vi "SwissSPAD Live.vi"() -> ()   [LabVIEW 2021]
uses:
  SwissSPAD Live_Internal Variables.ctl
  <vilib>/vision/Image Controls.llb/IMAQ Image.ctl
  SwissSPAD Live_Image ROI Information.ctl
  Phasor/Image Binning Options.ctl
  SwissSPAD Live_SSx PCB Version.ctl
  SwissSPAD Live_Q [Element].ctl
  SwissSPAD Live_Q Event List.ctl
  SwissSPAD Live_Windows List.ctl
  Sound/System Sounds List.ctl
  Image/Image Display to Clipboard Options.ctl
  Image/Image Display Palette Information.ctl
  Image/Image Display Palette Type.ctl
  SwissSPAD Live_Internal Data List.ctl
  SwissSPAD Live_Globals.vi
  D:/UCLA Thinkpad Google Drive/LabVIEW 2021 SP1/builds/SwissSPAD Live Distribution/Opal Kelly/C# Wrapper/v5.0.2/libFrontPanel-csharp.dll
  Opal Kelly/C# Wrapper/v5.0.2/libFrontPanel-csharp.dll
  Notebook/Notebook.lvlib
  Rich Text Box/Rich Text Box.lvlib
  Variant/Variant to Data/Variant to Data.lvlib
  Opal Kelly/C# Wrapper/okFrontPanelC#Wrapper.lvlib
panel:
  in  "Refresh":bool
  out "Top FPGA Status":bool caption="Top"
  out "Bottom FPGA Status":bool caption="Bot"
  out "Image":T1(plugin-control)
  out "Saving in progress":bool
  in  "Animated Busy Icon":bool=TRUE
  in  "Record Button":bool
  in  "Live Button":bool
  in  "Abort":bool
  out "Message":string
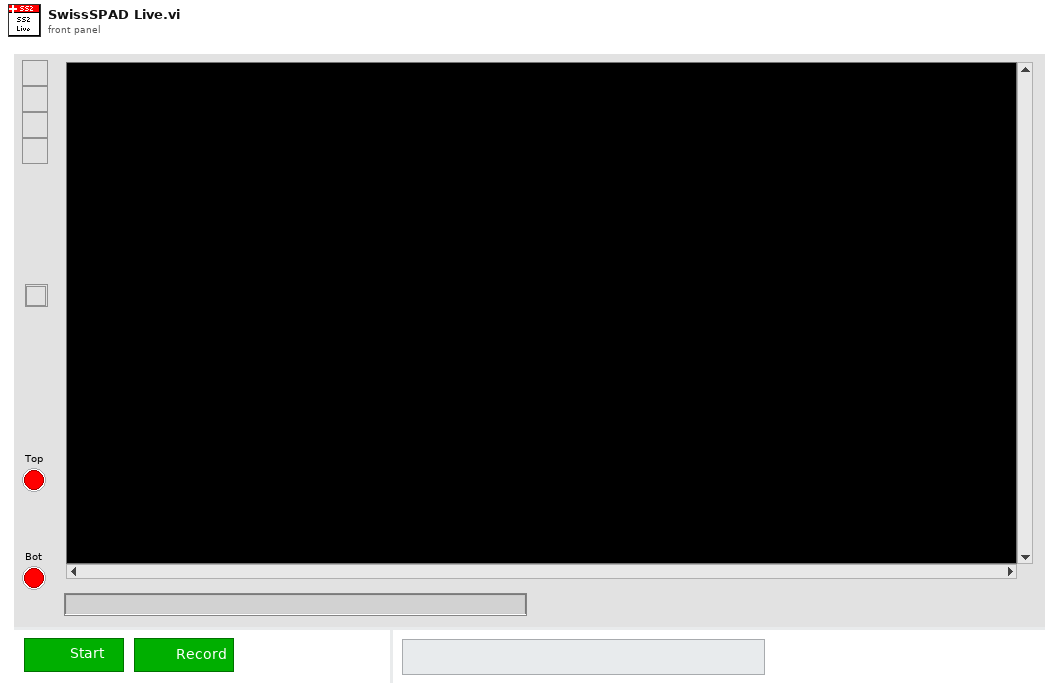
[diagram p1: front panel]
types:
  T1 = typedef "IMAQ Image.ctl" = refnum<image>
  T2 = typedef "SwissSPAD Live_Windows List.ctl" = enum16{"Settings Window", "Notebook Window", "Histogram Window", "About Window", "SS2 Live Window"}
  T3 = typedef "SwissSPAD Live_Q Event List.ctl" = enum16{"---- UI ----", "Idle", "Initialization", "Init FPGA(s)", "Init Top FPGA (deprecated)", "FPGA(s) Status", "Top FPGA Status (deprecated)", "Reset FPGA(s)", "Reset Top FPGA (deprecated)", "Refresh Display Image", "Quit", "---- DAQ ----", "Start Recording", "Start Live Acquisition", "Initialize Recording Mode", "Initialize FPGA (Live Mode)", "Get Image Set", "Get Single Image", "Update Image Display", "Stop Live Acquisition", "Stop Data Recording", "Stop Data Saving", "---- Image ----", "Copy Data to Clipboard", "Set Image Palette", "Save Displayed Image with Overlay", "Save Image Data as TIFF"}
  T4 = typedef "SwissSPAD Live_Q [Element].ctl" = cluster{"SwissSPAD Q Event":T3, "Data":variant}
  T5 = typedef "SwissSPAD Live_Internal Variables.ctl" = cluster{"okCFrontPanelDevices Refnum":refnum<k24>, "Bottom Device Refnum":refnum<k24>, "Display Image":T1, "# Live Images":i32, "relative s":dbl, "# Image Sets":i32, "Message":string, "Current Image Set":i32, "# Datasets in Series":i32, "Current Dataset":i32, "Live Mode":bool, "Recording Mode":bool, "Record Button":refnum<vi>, "\nLive Button":refnum<vi>, "SwissSPAD Live Gate Image Data Q Name":string, "Discard First Image":bool, "Image Information":T6, "Image Binning Options":T7, "Bottom FPGA Serial Number":string, "Detector PCB Version":T8, "# Acquisitions":u32, "10 bits":bool, "Top FPGA Serial Number":string, "Top Device Refnum":refnum<k24>}
  T6 = typedef "SwissSPAD Live_Image ROI Information.ctl" = cluster{"Save ROI Only":bool, "Left":u16, "Top":u16, "Right":u16, "Bottom":u16, "Use Current ROI":bool}
  T7 = typedef "Image Binning Options.ctl" = cluster{"Use Image Binning":bool, "X Bin":i32, "Y Bin":i32}
  T8 = typedef "SwissSPAD Live_SSx PCB Version.ctl" = enum16{"unknown", "SS2 PCB1", "SS2 PCB2", "SS3 PCB1"}
  T9 = typedef "System Sounds List.ctl" = enum16{"Alarm01", "Alarm02", "Alarm03", "Alarm04", "Alarm05", "Alarm06", "Alarm07", "Alarm08", "Alarm09", "Alarm10", "chimes", "chord", "ding", "notify", "recycle", "Ring01", "Ring02", "Ring03", "Ring04", "Ring05", "Ring06", "Ring07", "Ring08", "Ring09", "Ring10", "ringout", "Speech Off", "Speech On", "Speech Sleep", "tada", "Windows Background", "Windows Balloon", "Windows Battery Critical", "Windows Battery Low", "Windows Critical Stop", "Windows Default", "Windows Ding", "Windows Error", "Windows Exclamation", "Windows Feed Discovered", "Windows Foreground", "Windows Hardware Fail", "Windows Hardware Insert", "Windows Hardware Remove", "Windows Information Bar", "Windows Logoff Sound", "Windows Logon", "Windows Menu Command", "Windows Message Nudge", "Windows Minimize", "Windows Navigation Start", "Windows Notify Calendar", "Windows Notify Email", "Windows Notify Messaging", "Windows Notify System Generic", "Windows Notify", "Windows Pop-up Blocked", "Windows Print complete", "Windows Proximity Connection", "Windows Proximity Notification", "Windows Recycle", "Windows Restore", "Windows Ringin", "Windows Ringout", "Windows Shutdown", "Windows Startup", "Windows Unlock", "Windows User Account Control"}
  T10 = typedef "Image Display to Clipboard Options.ctl" = cluster{"Include Overlay (T)":bool, "Image Only (T)":bool}
  T11 = cluster{"CtlRef":refnum<vi>, "Image to Clipboard Options":T10}
  T12 = typedef "Image Display Palette Information.ctl" = cluster{"Palette Name [# Colors,int?,inv?]":string, "Palette Type":T13, "Palette Colors":u32[], "Interpolate?":bool}
  T13 = typedef "Image Display Palette Type.ctl" = u32
  T14 = typedef "SwissSPAD Live_Init Communication Outcome.ctl" = cluster{"Bottom FPGA Found":bool, "Top FPGA Found":bool, "# Orphan FPGAs":i32, "Orphaned FPGA S/N":string[]}
  T15 = typedef "Rich Text Box.lvlib/Text Formatting.ctl" = cluster{"Font":string, "Text Color":T16, "Text Background Color":T16, "Text Style":enum16{"Regular", "Bold", "Italic", "Underline", "Strikeout"}, "Font Size (Points)":dbl, "Text Alignment":i32}
  T16 = typedef "Rich Text Box.lvlib/Text Colors.ctl" = enum16{"Unchanged", "Black", "Blue", "Brown", "Gray", "Green", "Orange", "Pink", "Red", "White"}
  T17 = typedef "Save File Format.ctl" = enum16{"PNG", "JPEG", "BMP"}
  T18 = typedef "SwissSPAD Live_Internal Data List.ctl" = enum16{"Number of pending file saving tasks", "File Saving Tasks Information", "Current Image ROI Information", "# FPGA Reset Attempts", "Histogram Cursor Locations", "Histogram Window is Open"}
  T19 = cluster{"Global Rectangle":i32[], "Contours":cluster{"Contour Type":u32, "ROI Type":u32, "Points":i32[]}[]}
  T20 = typedef "SwissSPAD Live_File Saving Task Information.ctl" = cluster{"File Path::n":string, "# Saved Images":i32, "# Images (Total)":i32, "File Size (Bytes)":i64}
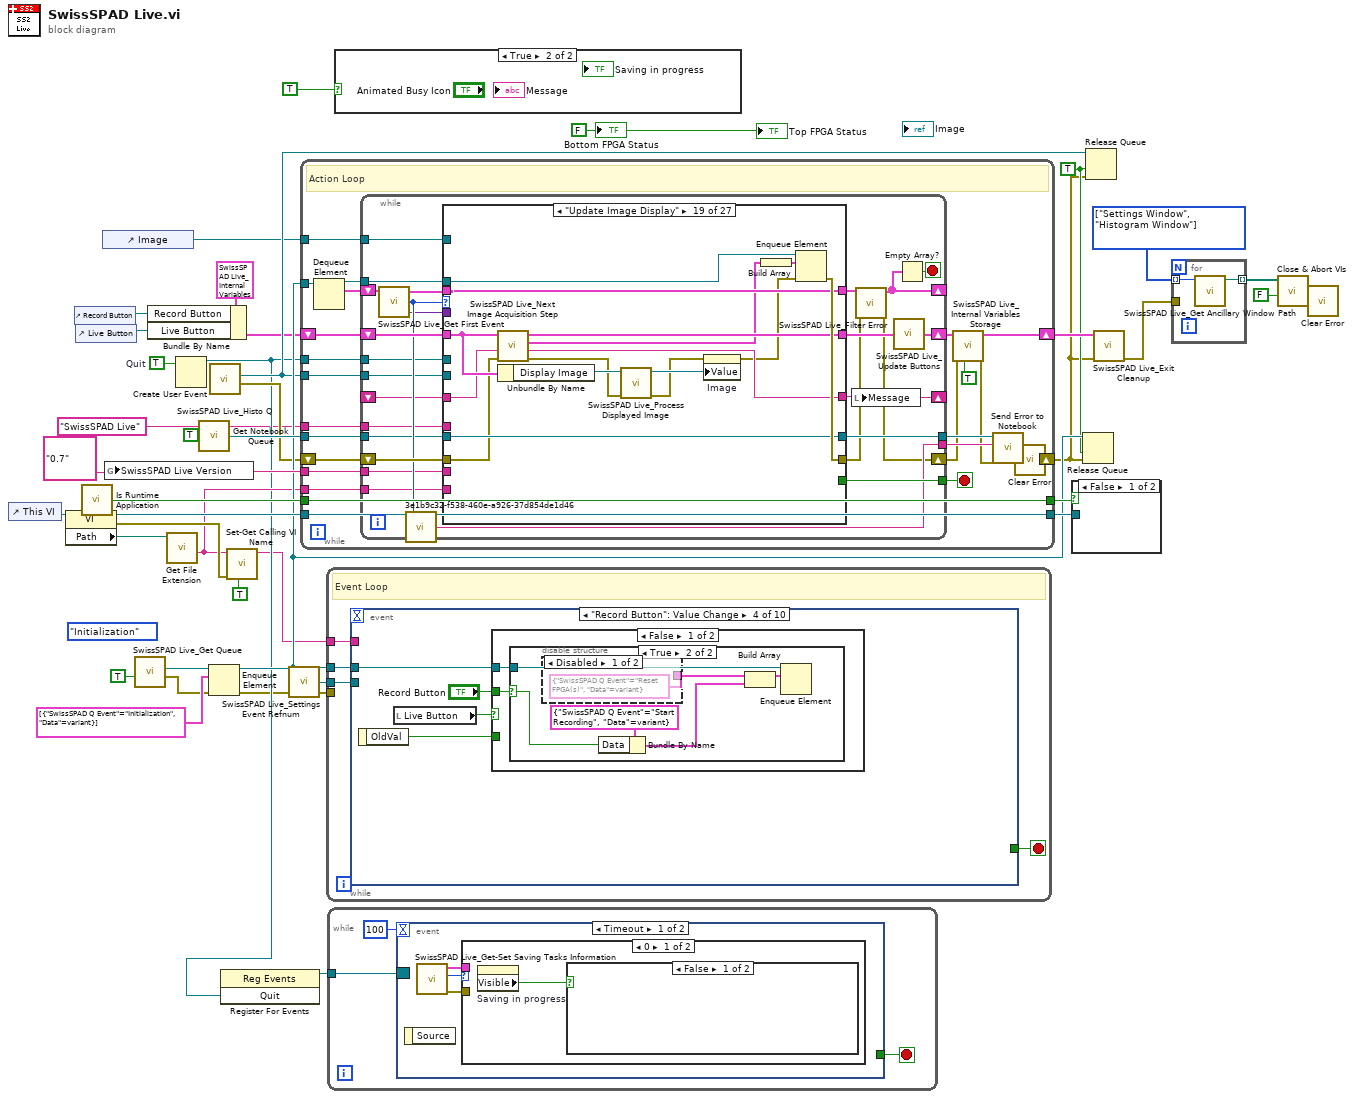
[diagram p0: block diagram]
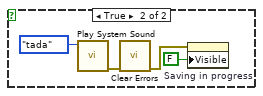
[diagram p2: hidden frame]
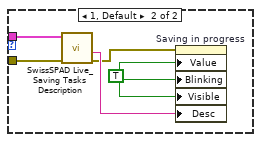
[diagram p3: hidden frame]
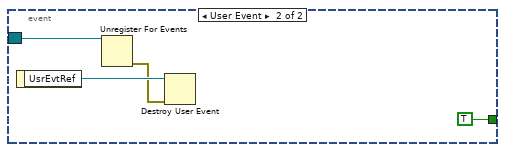
[diagram p4: hidden frame]
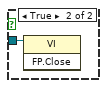
[diagram p6: hidden frame]
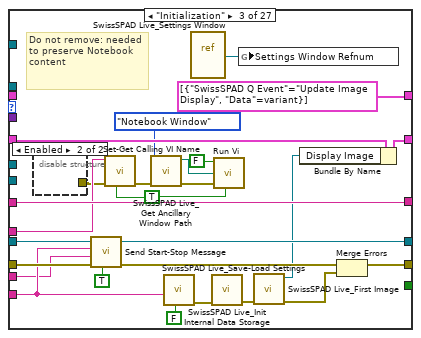
[diagram p9: hidden frame]
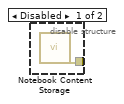
[diagram p10: hidden frame]
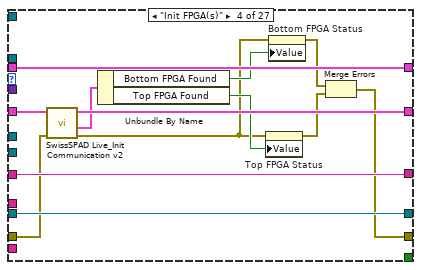
[diagram p11: hidden frame]
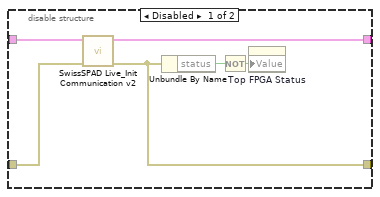
[diagram p13: hidden frame]
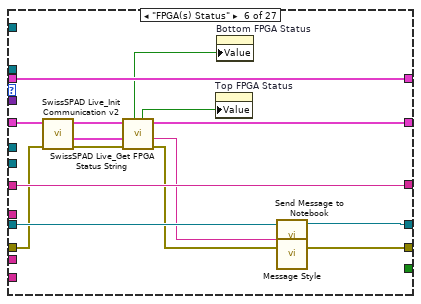
[diagram p14: hidden frame]
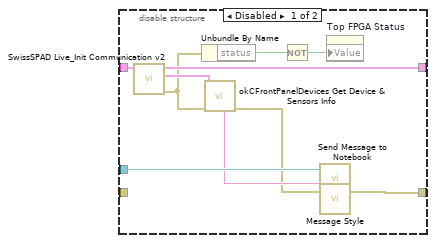
[diagram p16: hidden frame]
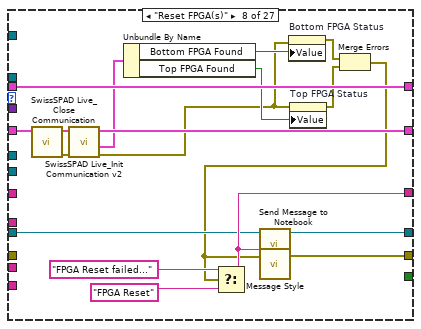
[diagram p17: hidden frame]
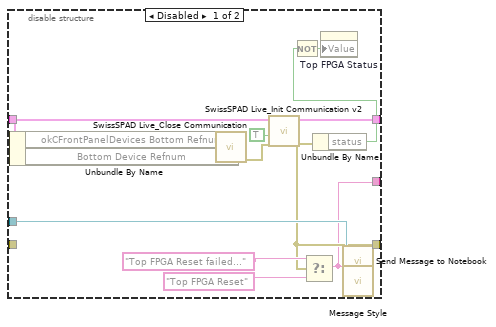
[diagram p19: hidden frame]
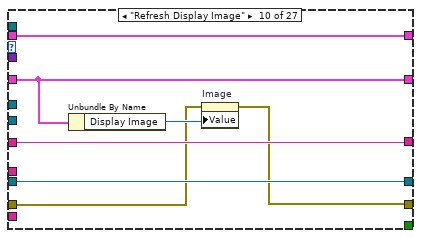
[diagram p20: hidden frame]
diagram:
  w6 = T2[] [enum."Settings Window", enum."Histogram Window"] items=["Settings Window", "Notebook Window", "Histogram Window", "About Window", "SS2 Live Window"] ("Array")
  (unwired) SwissSPAD_Live_Q_Event_List."Initialization" ("SwissSPAD Q Event")
  w7 = FALSE ("FPGA Status")
  w22 = TRUE  # Quit
  w25 = TRUE ("force destroy? (F)")
  w30 = "0.7" ("SS2 Live Version")
  n1 = control-ref of="This VI"() -> (w40:refnum<vi>)
  n2 = property class="VI"(reference=w40) -> (reference out=w37:refnum<vi>, error out=w36:errorcluster, "Path"=w26:path)  [unwired: 1 in]
  n3 = control-ref of="Record Button"() -> (w12:refnum<vi>)
  n4 = control-ref of="Live Button"() -> (w13:refnum<vi>)
  n5 = call "Is Runtime Application.vi"() -> ("Runtime ?"=w42:bool)  [unwired: 8 in, 1 out]
  n6 = control-ref of="Image"() -> (w15:refnum<vi>)
  n7 = global write "SwissSPAD Live_Globals.vi" "SwissSPAD Live Version"(w30) -> ()
  n8 = call "SwissSPAD Live_Get Queue.vi"("create if not found? (F)"=TRUE) -> ("error out"=w9:errorcluster, "SwissSPAD Queue"=w10:refnum<queue>)  [unwired: 9 in]
  n9 = Bundle By Name(cluster=T5 {"okCFrontPanelDevices Refnum"=refnum, "Bottom Device Refnum"=refnum, "Display Image"=refnum, "# Live Images"=0, "relative s"=nan, "# Image Sets"=0, "Message"="", "Current Image Set"=0, "# Datasets in Series"=0, "Current Dataset"=0, "Live Mode"=FALSE, "Recording Mode"=FALSE, "Record Button"=refnum, "\nLive Button"=refnum, "SwissSPAD Live Gate Image Data Q Name"="SS2 Live Gate Data Q", "Discard First Image"=FALSE, "Image Information"={"Save ROI Only"=FALSE, "Left"=0, "Top"=0, "Right"=0, "Bottom"=0, "Use Current ROI"=FALSE}, "Image Binning Options"={"Use Image Binning"=FALSE, "X Bin"=1, "Y Bin"=1}, "Bottom FPGA Serial Number"="", "Detector PCB Version"=enum."unknown", "# Acquisitions"=0, "10 bits"=FALSE, "Top FPGA Serial Number"="", "Top Device Refnum"=refnum}, "Record Button"=w12, "Live Button"=w13) -> (w14:T5)
  n10 = call <vilib>:"Get File Extension.vi"("file"=w26) -> ("filename without extension"=w27:string)  [unwired: 6 in, 4 out]
  n11 = Create User Event(user event datatype=w22) -> (user event=w20:refnum<user-event>)  [unwired: 1 in, 1 out]
  n12 = call "Get Notebook Queue.vi"("create if not found? (T)"=TRUE ("create if not found? (F)")) -> ("Notebook Queue"=w31:refnum<queue>)  [unwired: 8 in]
  n13 = Enqueue Element(queue=w10, element=T4[] [{"SwissSPAD Q Event"=enum."Initialization", "Data"=variant}], error in (no error)=w9) -> (queue out=w29:refnum<queue>, error out=w19:errorcluster)  [unwired: 1 in, 1 out]
  n14 = call "SwissSPAD Live_Histo Q.vi"() -> ("error out"=w24:errorcluster, "SS2 Live Histo Q"=w23:refnum<queue>)  [unwired: 6 in]
  n15 = register-events(w20) -> (reference out=w21:refnum<event-registration>)  [unwired: 2 in, 1 out]
  n16 = call "Set-Get Calling VI Name.vi"("Set/Get (F)"=TRUE, "Error In"=w36, "Calling VI Name"=w27) -> ("Calling VI Name"=w16:string)  [unwired: 7 in, 1 out]
  n17 = call "SwissSPAD Live_Settings Event Refnum.vi"("Error In"=w19) -> ("Settings Event Refnum"=w17:refnum<user-event>, "Error Out"=w18:errorcluster)  [unwired: 7 in]
  n18 = while {
    tunnel: w29 -> [w66]
    tunnel: w42 -> [w61]
    tunnel: [w61] -> w41
    tunnel: w37 -> [w60]
    tunnel: [w60] -> w39
    shift-right: [w54] -> w5
    shift-left: w24 -> [w63]
    shift-right: [w46] -> w33
    shift-left: w14 -> [w59]
    tunnel: w31 -> [w57]
    tunnel: w30 -> [w52]
    tunnel: w27 -> [w51]
    tunnel: w23 -> [w50]
    tunnel: w20 -> [w49]
    tunnel: w15 -> [w48]
    tunnel: "SwissSPAD Live" ("Calling VI Name") -> [w47]
    stop <- w64 stop-if-true
    # "Action Loop"
    n19 = Dequeue Element(queue=w66) -> (queue out=w62:refnum<queue>, element=w65:T4[])  [unwired: 2 in, 2 out]
    n20 = while {
      tunnel: [w92] -> w64
      tunnel: w62 -> [w90]
      shift-right: [w68] -> w44
      shift-left: w63 -> [w91]
      shift-right: [w67] -> _
      shift-left: w65 -> [w89]
      shift-right: [w76] -> w58
      shift-left: w59 -> [w86]
      tunnel: w57 -> [w83]
      tunnel: [w71] -> w56
      tunnel: [w84] -> w53
      tunnel: w52 -> [w82]
      tunnel: w51 -> [w81]
      shift-right: [w80] -> _
      shift-left: _ -> [w79]
      tunnel: w50 -> [w77]
      tunnel: w49 -> [w75]
      tunnel: w48 -> [w73]
      tunnel: w47 -> [w72]
      stop <- w87 stop-if-true
      n21 = call "SwissSPAD Live_Get First Event.vi"("SS2 Q Element"=w89) -> ("Data"=w78:variant, "SS2 Q Event"=w85:T3, "SS2 Q Elements"=w88:T4[])  [unwired: 2 in]
      n22 = call "3e1b9c32-f538-460e-a926-37d854de1d46.vi"("Enum"=w85) -> ("String"=w84:string)
      n23 = case shown="\"Update Image Display\"" w85 {
        tunnel: [_ _ _ _ _ _ _ _ _ _ w252 _ _ _ _ _ _ _ _ _ _ _ _ _ _ _ _] -> w92
        tunnel: w91 -> [w97 w102 w121 w136 w143 w157 w173 _ w212 w236 w253 w266 w271 w292 w303 w316 _ w356 w367 w378 _ w404 w412 w420 w425 w442 w479]
        tunnel: w90 -> [_ _ _ _ _ _ _ _ _ _ _ _ w276 w295 w307 w320 w348 w359 w372 w384 w397 _ _ _ _ _ _]
        tunnel: [w97 w102 w126 w129 w142 w169 w177 w202 w214 w235 w261 w266 w275 w286 w296 w319 w339 w353 w375 w382 w387 w401 w412 w414 w426 w447 w484] -> w70
        tunnel: w88 -> [w96 w101 _ w141 w148 w172 w179 w211 w218 w241 _ w265 w274 w293 w305 w318 w346 w358 w374 _ _ w407 w411 w424 w439 w451 w488]
        tunnel: [w96 w101 T4[] [{"SwissSPAD Q Event"=enum."Update Image Display", "Data"=variant}] ("SS2 Q Elements") w141 w148 w172 w179 w211 w218 w241 _ w265 w274 w293 w305 w318 w346 w358 w374 _ _ w407 w411 w424 w439 w451 w488] -> w69
        tunnel: w86 -> [w93 w100 w127 w138 w145 w167 w175 w200 w216 w238 w244 w262 w273 w291 w304 w311 w343 w355 w370 w379 w386 w406 w408 w419 w430 w450 w486]
        tunnel: [w93 w100 w115 w137 w144 w163 w174 w210 w217 w238 w243 w262 w273 w289 w300 w310 w342 w351 w369 w377 w395 w406 w408 w419 w430 w450 w486] -> w74
        tunnel: w77 -> [_ _ _ _ _ _ _ _ _ _ w256 _ _ _ _ _ _ _ _ _ _ _ _ _ _ _ _]
        tunnel: w83 -> [w95 w99 w123 w140 w147 w168 w176 w203 w215 w240 w254 w264 w270 w290 w301 w315 w341 w357 w373 w381 w393 w402 w410 w423 w438 w440 w483]
        tunnel: w82 -> [_ _ w119 _ _ _ _ _ _ _ w248 _ _ _ _ _ _ _ _ _ _ _ _ _ _ _ _]
        tunnel: w81 -> [_ _ w120 _ _ _ _ _ _ _ w249 _ _ _ _ _ _ _ _ _ _ _ _ _ _ _ _]
        tunnel: [w95 w99 w123 w140 w147 w164 w176 w204 w215 w240 w254 w264 w270 w290 w301 w315 w335 w357 w373 w381 w393 w398 w410 w423 w438 w440 w475] -> w71
        tunnel: [w94 w98 w125 w139 w146 w171 w178 w205 w213 w239 w259 w263 w272 w287 w297 w313 "" ("Message") w349 w366 "Live Mode stopped" ("Message") "Data Recording stopped" ("Message") w399 w409 w422 w437 w449 w487] -> w80
        tunnel: w79 -> [w94 w98 w125 w139 w146 w171 w178 _ _ w239 w259 w263 _ _ _ _ _ _ w365 _ _ _ w409 w422 w437 w449 w487]
        tunnel: w78 -> [_ _ _ _ _ _ _ _ _ _ _ _ _ _ _ w309 _ _ _ _ _ _ _ w421 w432 _ _]
        tunnel: w75 -> [_ _ _ _ _ _ _ _ _ _ w247 _ _ _ _ _ _ _ _ _ _ _ _ _ _ _ _]
        tunnel: w73 -> [_ _ _ _ _ _ _ _ _ _ _ _ _ _ _ _ _ _ _ _ _ _ _ _ w427 w448 _]
        tunnel: w72 -> [_ _ w109 _ _ _ _ _ _ _ _ _ _ _ _ _ _ _ _ _ _ _ _ _ _ _ _]
        frame "---- UI ----" {
        }
        frame "Idle", Default {
        }
        frame "Initialization" {
          w107 = TRUE ("Start Hidden? (F)")
          # "Do not remove: needed to preserve Notebook content"
          n24 = disable-structure shown="Enabled" {
            disable-tunnel: [w128 _] -> w108
            frame Disabled {
              n25 = call "Notebook Content Storage.vi"() -> ("Error Out"=w128:errorcluster)  [unwired: 10 in, 1 out]
            }
            frame Enabled {
            }
          }
          n26 = call "Send Start-Stop Message.vi"("Start(T)/Stop(F)"=TRUE ("Start(F)/Stop(T)"), "Error In"=w121, "Version number"=w119, "Software Name"=w120, "Notebook Queue"=w123) -> ("Error Out"=w122:errorcluster)  [unwired: 6 in]
          n27 = call "Set-Get Calling VI Name.vi"("Set/Get (F)"=w107, "Error In"=w108, "Calling VI Name"=w109) -> ("Error Out"=w110:errorcluster)  [unwired: 7 in, 1 out]
          n28 = call "SwissSPAD Live_Get Ancillary Window Path.vi"("Error In"=w110, "SS2 Live Windows"=SwissSPAD_Live_Windows_List."Notebook Window") -> ("Error Out"=w113:errorcluster, "VI Path"=w112:path)  [unwired: 8 in]
          n29 = call "SwissSPAD Live_Save-Load Settings.vi"("Load(F)/Save (T)"=FALSE, "App Name"=w120) -> ("Error Out"=w106:errorcluster)  [unwired: 8 in, 1 out]
          n30 = vi-ref "SwissSPAD Live_Settings Window.vi"() -> (w124:refnum<vi>)
          n31 = call "SwissSPAD Live_Init Internal Data Storage.vi"("Error In"=w106) -> ("Error Out"=w104:errorcluster)  [unwired: 10 in]
          n32 = call "Run Vi.vi"("Bring To Front (T)"=FALSE, "VI Path"=w112, "error in (no error)"=w113, "Start Hidden? (F)"=w107) -> ()  [unwired: 4 in, 2 out]
          n33 = global write "SwissSPAD Live_Globals.vi" "Settings Window Refnum"(w124) -> ()
          n34 = call "SwissSPAD Live_First Image.vi"("error in"=w104) -> ("error out"=w103:errorcluster, "Image"=w114:T1)  [unwired: 9 in]
          n35 = Bundle By Name(cluster=w127, "Display Image"=w114) -> (w115:T5)
          n36 = Merge Errors(w122, w103) -> (w126:errorcluster)
        }
        frame "Init FPGA(s)" {
          n37 = call "SwissSPAD Live_Init Communication v2.vi"("Error In"=w136, "SwissSPAD Live Internal Variables in"=w138) -> ("Error Out"=w132:errorcluster, "Init Communication Outcome"=w135:T14, "SwissSPAD Live Internal Variables out"=w137:T5)  [unwired: 7 in]
          n38 = Unbundle By Name(w135) -> ("Bottom FPGA Found"=w134:bool, "Top FPGA Found"=w133:bool)
          n39 = property on="Top FPGA Status" class="Bool (strict)"(error in=w132, "Value"=w133) -> (error out=w130:errorcluster)  [unwired: 1 in, 1 out]
          n40 = property on="Bottom FPGA Status" class="Bool (strict)"(error in=w132, "Value"=w134) -> (error out=w131:errorcluster)  [unwired: 1 in, 1 out]
          n41 = Merge Errors(w131, w130) -> (w129:errorcluster)
        }
        frame "Init Top FPGA (deprecated)" {
          n42 = disable-structure shown="Enabled" {
            disable-tunnel: w145 -> [w154 w156]
            disable-tunnel: [w153 w156] -> w144
            disable-tunnel: w143 -> [w152 w155]
            disable-tunnel: [w151 w155] -> w142
            frame Disabled {
              n43 = call "SwissSPAD Live_Init Communication v2.vi"("Error In"=w152, "SwissSPAD Live Internal Variables in"=w154) -> ("Error Out"=w151:errorcluster, "SwissSPAD Live Internal Variables out"=w153:T5)  [unwired: 7 in, 1 out]
              n44 = Unbundle By Name(w151) -> ("status"=w150:bool)
              n45 = Not(x=w150) -> (.not. x?=w149:bool)
              n46 = property on="Top FPGA Status" class="Bool (strict)"("Value"=w149) -> ()  [unwired: 2 in, 2 out]
            }
            frame Enabled {
            }
          }
        }
        frame "FPGA(s) Status" {
          n47 = call "SwissSPAD Live_Init Communication v2.vi"("Error In"=w157, "SwissSPAD Live Internal Variables in"=w167) -> ("Error Out"=w165:errorcluster, "Init Communication Outcome"=w161:T14, "SwissSPAD Live Internal Variables out"=w160:T5)  [unwired: 7 in]
          n48 = call "SwissSPAD Live_Get FPGA Status String.vi"("error in (no error)"=w165, "Init Communication Outcome"=w161, "SwissSPAD Live Internal Variables in"=w160) -> ("error out"=w166:errorcluster, "Device Info String"=w162:string, "SwissSPAD Live Internal Variables out"=w163:T5, "Top FPGA Status"=w158:bool, "Bottom FPGA Status"=w159:bool)  [unwired: 4 in]
          n49 = property on="Top FPGA Status" class="Bool (strict)"("Value"=w158) -> ()  [unwired: 2 in, 2 out]
          n50 = property on="Bottom FPGA Status" class="Bool (strict)"("Value"=w159) -> ()  [unwired: 2 in, 2 out]
          n51 = call "Message Style.vi"() -> ("Message Formatting"=w170:T15)
          n52 = call "Send Message to Notebook.vi"("Text Formatting"=w170, "Error In"=w166, "Message"=w162, "Notebook Queue"=w168) -> ("Error Out"=w169:errorcluster, "Notebook Queue"=w164:refnum<queue>)  [unwired: 4 in]
        }
        frame "Top FPGA Status (deprecated)" {
          n53 = disable-structure shown="Enabled" {
            disable-tunnel: [w189 w191] -> w177
            disable-tunnel: w176 -> [w188 _]
            disable-tunnel: w175 -> [w187 w192]
            disable-tunnel: [w183 w192] -> w174
            disable-tunnel: w173 -> [_ w191]
            frame Disabled {
              n54 = call "SwissSPAD Live_Init Communication v2.vi"("SwissSPAD Live Internal Variables in"=w187) -> ("Error Out"=w182:errorcluster, "Init Communication Outcome"=w186:T14, "SwissSPAD Live Internal Variables out"=w183:T5)  [unwired: 8 in]
              n55 = Unbundle By Name(w182) -> ("status"=w181:bool)
              n56 = call "okCFrontPanelDevices Get Device & Sensors Info.vi"("error in (no error)"=w182, "okCFrontPanel Device Refnum"=w186) -> ("error out"=w184:errorcluster, "Device Info String"=w185:string)  [unwired: 5 in, 3 out]
              n57 = Not(x=w181) -> (.not. x?=w180:bool)
              n58 = call "Message Style.vi"() -> ("Message Formatting"=w190:T15)
              n59 = call "Send Message to Notebook.vi"("Text Formatting"=w190, "Error In"=w184, "Message"=w185, "Notebook Queue"=w188) -> ("Error Out"=w189:errorcluster)  [unwired: 7 in]
              n60 = property on="Top FPGA Status" class="Bool (strict)"("Value"=w180) -> ()  [unwired: 2 in, 2 out]
            }
            frame Enabled {
            }
          }
        }
        frame "Reset FPGA(s)" {
          n61 = call "SwissSPAD Live_Close Communication.vi"("SwissSPAD Live Internal Variables"=w200) -> ("Error Out"=w209:errorcluster, "SwissSPAD Live Internal Variables"=w201:T5)  [unwired: 9 in]
          n62 = call "SwissSPAD Live_Init Communication v2.vi"("Error In"=w209, "SwissSPAD Live Internal Variables in"=w201) -> ("Error Out"=w196:errorcluster, "Init Communication Outcome"=w199:T14, "SwissSPAD Live Internal Variables out"=w210:T5)  [unwired: 7 in]
          n63 = Unbundle By Name(w199) -> ("Bottom FPGA Found"=w198:bool, "Top FPGA Found"=w197:bool)
          n64 = call "Message Style.vi"() -> ("Message Formatting"=w208:T15)
          n65 = property on="Bottom FPGA Status" class="Bool (strict)"(error in=w196, "Value"=w198) -> (error out=w195:errorcluster)  [unwired: 1 in, 1 out]
          n66 = property on="Top FPGA Status" class="Bool (strict)"(error in=w196, "Value"=w197) -> (error out=w193:errorcluster)  [unwired: 1 in, 1 out]
          n67 = Merge Errors(w195, w193) -> (w194:errorcluster)
          n68 = Select(t="FPGA Reset failed...", s=w194, f="FPGA Reset" ("UI Message")) -> (s? t:f=w205:string)
          n69 = call "Send Message to Notebook.vi"("Text Formatting"=w208, "Error In"=w194, "Message"=w205, "Notebook Queue"=w203) -> ("Error Out"=w202:errorcluster, "Notebook Queue"=w204:refnum<queue>)  [unwired: 4 in]
        }
        frame "Reset Top FPGA (deprecated)" {
          n70 = disable-structure shown="Enabled" {
            disable-tunnel: [w232 w234] -> w217
            disable-tunnel: w216 -> [w229 w234]
            disable-tunnel: w215 -> [w225 _]
            disable-tunnel: [w222 w233] -> w214
            disable-tunnel: [w219 _] -> w213
            disable-tunnel: w212 -> [_ w233]
            frame Disabled {
              n71 = Unbundle By Name(w229) -> ("okCFrontPanelDevices Bottom Refnum"=w231:refnum<k24>, "Bottom Device Refnum"=w230:refnum<k24>)
              n72 = call "SwissSPAD Live_Close Communication.vi"(10:w230, "SwissSPAD Live Internal Variables"=w231) -> ("Error Out"=w228:errorcluster)  [unwired: 8 in, 1 out]
              n73 = call "SwissSPAD Live_Init Communication v2.vi"("Init Communication Outcome"=TRUE ("Reset FPGA"), "Error In"=w228, "SwissSPAD Live Internal Variables in"=w229) -> ("Error Out"=w222:errorcluster, "SwissSPAD Live Internal Variables out"=w232:T5)  [unwired: 7 in]
              n74 = Select(t="Top FPGA Reset failed...", s=w222, f="Top FPGA Reset" ("UI Message")) -> (s? t:f=w219:string)
              n75 = Unbundle By Name(w222) -> ("status"=w221:bool)
              n76 = Not(x=w221) -> (.not. x?=w220:bool)
              n77 = property on="Top FPGA Status" class="Bool (strict)"("Value"=w220) -> ()  [unwired: 2 in, 2 out]
              n78 = call "Message Style.vi"() -> ("Message Formatting"=w226:T15)
              n79 = call "Send Message to Notebook.vi"("Text Formatting"=w226, "Message"=w219, "Notebook Queue"=w225) -> ()  [unwired: 8 in, 1 out]
            }
            frame Enabled {
            }
          }
        }
        frame "Refresh Display Image" {
          n80 = Unbundle By Name(w238) -> ("Display Image"=w237:T1)
          n81 = property on="Image" class="ImageControl"(error in=w236, "Value"=w237) -> (error out=w235:errorcluster)  [unwired: 1 in, 1 out]
        }
        frame "Quit" {
          w252 = TRUE
          # "quits Histogram Window"
          n82 = Generate User Event(user event=w247, event data cluster=TRUE ("event data")) -> ()  [unwired: 2 in, 2 out]
          n83 = call "SwissSPAD Live_Save-Load Settings.vi"("Load(F)/Save (T)"=w252, "Error In"=w253, "App Name"=w249) -> ("Error Out"=w260:errorcluster)  [unwired: 7 in, 1 out]
          n84 = call "Send Start-Stop Message.vi"("Start(T)/Stop(F)"=FALSE, "Error In"=w253, "Version number"=w248, "Software Name"=w249, "Notebook Queue"=w254) -> ("Error Out"=w250:errorcluster)  [unwired: 6 in]
          n85 = Enqueue Element(queue=w256, element=u16[][] [], timeout in ms (-1)=10, error in (no error)=w253) -> (error out=w251:errorcluster)  [unwired: 2 out]
          n86 = call "Clear Error.vi"("Error In"=w251) -> ("no Error Out"=w242:errorcluster)  [unwired: 8 in]
          n87 = call "Delete Notebook Backup on Quit.vi"("Main VI Name"=w249) -> ("Error Out"=w258:errorcluster)  [unwired: 10 in]
          n88 = call "SwissSPAD Live_Clear Internal Variables.vi"("SS2 Live Internal Variables in"=w244) -> ("SS2 Live Internal Variables"=w243:T5)  [unwired: 10 in]
          n89 = Merge Errors(w242, w260, w250, w258) -> (w261:errorcluster)
        }
        frame "---- DAQ ----" {
        }
        frame "Start Live Acquisition" {
          n90 = property on="Top FPGA Status" class="Bool (strict)"() -> ("Value"=w267:bool)  [unwired: 2 in, 2 out]
          n91 = property on="Bottom FPGA Status" class="Bool (strict)"() -> ("Value"=w269:bool)  [unwired: 2 in, 2 out]
          n92 = Compound Arithmetic op=OR(w267, w269) -> (w268:bool)
          n93 = case shown="True" w268 {
            tunnel: w276 -> [_ w283]
            tunnel: [w278 w280] -> w275
            tunnel: w271 -> [w278 w284]
            tunnel: [w277 "Live Acquisition..." ("Message")] -> w272
            frame False {
              w277 = "No active FPGA!" ("message")
              n94 = call "System Error Sound.vi"() -> ()  [unwired: 27 in, 1 out]
              n95 = One Button Dialog(message=w277) -> ()  [unwired: 1 in, 1 out]
            }
            frame True {
              n96 = call "Show Animated Busy Icon with Message.vi"("Error In"=w284) -> ("Error Out"=w281:errorcluster)  [unwired: 10 in]
              n97 = Build Array(T4 {"SwissSPAD Q Event"=enum."Initialize FPGA (Live Mode)", "Data"=variant} ("SS2 Live Atomic Action")) -> (w282:T4[])
              n98 = Enqueue Element(queue=w283, element=w282, error in (no error)=w281) -> (error out=w280:errorcluster)  [unwired: 1 in, 2 out]
            }
          }
        }
        frame "Initialize FPGA (Live Mode)" {
          n99 = call "SwissSPAD Live_Init Live Acquisition.vi"("error in (no error)"=w292, "SwissSPAD Live Internal Variables in"=w291) -> ("error out"=w286:errorcluster, "Message"=w287:string, "SwissSPAD Live Atomic Action"=w288:T4, "SwissSPAD Live Internal Variables out"=w289:T5)  [unwired: 6 in]
          n100 = Build Array(w288) -> (w294:T4[])
          n101 = Enqueue Element(queue=w295, element=w294) -> ()  [unwired: 2 in, 3 out]
        }
        frame "Get Single Image" {
          n102 = call "SwissSPAD Live_Get Single Image.vi"("error in (no error)"=w303, "SwissSPAD Live Internal Variables"=w304) -> ("error out"=w299:errorcluster, "SwissSPAD Live Internal Variables out"=w302:T5)  [unwired: 8 in]
          n103 = call "SwissSPAD Live_Live Image Message.vi"("error in (no error)"=w299, "SS2 Live Internal Variables"=w302) -> ("error out"=w296:errorcluster, "Message"=w297:string, "SS2 Live Atomic Action"=w298:T4, "SS2 Live Internal Variables"=w300:T5)  [unwired: 6 in]
          n104 = Build Array(w298) -> (w306:T4[])
          n105 = Enqueue Element(queue=w307, element=w306) -> ()  [unwired: 2 in, 3 out]
        }
        frame "Start Recording" {
          n106 = call "Variant to Boolean.vi"("Variant"=w309) -> ("Value"=w308:bool)  [unwired: 8 in]
          n107 = call "SwissSPAD Live_Pre-Recording Checks.vi"("error in (no error)"=w316, "Init Series?"=w308, "SwissSPAD Live Internal Variables in"=w311) -> ("error out"=w317:errorcluster, "Message"=w312:string, "Ready?"=w314:bool, "SwissSPAD Live Internal Variables out"=w310:T5, "Verbose Message"=w313:string)  [unwired: 4 in]
          n108 = case shown="True" w314 {
            tunnel: w320 -> [_ w324]
            tunnel: [w322 w323] -> w319
            tunnel: w317 -> [w322 w325]
            tunnel: w312 -> [w321 _]
            frame False {
              n109 = One Button Dialog(message=w321) -> ()  [unwired: 1 in, 1 out]
            }
            frame True {
              n110 = case shown="No Error" w325 {
                selector: w325 -> [w330 w334]
                tunnel: w324 -> [w329 w333]
                tunnel: [w326 w334] -> w323
                frame No Error {
                  n111 = call "Show Animated Busy Icon with Message.vi"("Error In"=w330) -> ("Error Out"=w327:errorcluster)  [unwired: 10 in]
                  n112 = Build Array(T4 {"SwissSPAD Q Event"=enum."Initialize Recording Mode", "Data"=variant} ("SS2 Live Atomic Action")) -> (w328:T4[])
                  n113 = Enqueue Element(queue=w329, element=w328, error in (no error)=w327) -> (error out=w326:errorcluster)  [unwired: 1 in, 2 out]
                }
                frame Error {
                  n114 = Enqueue Element(queue=w333, element=T4[] [{"SwissSPAD Q Event"=enum."Stop Data Recording", "Data"=variant}]) -> ()  [unwired: 2 in, 3 out]
                }
              }
            }
          }
        }
        frame "Initialize Recording Mode" {
          n115 = call "SwissSPAD Live_Init Recording.vi"("SwissSPAD Live Internal Variables in"=w343) -> ("Error Out"=w336:errorcluster, "Notebook Message"=w338:string, "SwissSPAD Live Internal Variables out"=w342:T5)  [unwired: 8 in]
          n116 = Build Array(T4 {"SwissSPAD Q Event"=enum."Get Image Set", "Data"=variant} ("SS2 Live Queue Element Array")) -> (w347:T4[])
          n117 = Enqueue Element(queue=w348, element=w347, error in (no error)=w336) -> (error out=w340:errorcluster)  [unwired: 1 in, 2 out]
          n118 = call "Message Style.vi"() -> ("Message Formatting"=w337:T15)
          n119 = call "Send Message to Notebook.vi"("Text Formatting"=w337, "Error In"=w340, "Message"=w338, "Notebook Queue"=w341) -> ("Error Out"=w339:errorcluster, "Notebook Queue"=w335:refnum<queue>)  [unwired: 4 in]
        }
        frame "Get Image Set" {
          n120 = call "SwissSPAD Live_Get Single Image Set.vi"("error in (no error)"=w356, "SwissSPAD Live Internal Variables"=w355) -> ("error out"=w354:errorcluster, "SwissSPAD Live Internal Variables out"=w352:T5)  [unwired: 8 in]
          n121 = call "SwissSPAD Live_Get Next Series Step.vi"("error in (no error)"=w354, "SwissSPAD Live Internal Variables in"=w352) -> ("Error Out"=w353:errorcluster, "Message out"=w349:string, "SwissSPAD Live Atomic Action"=w350:T4[], "SwissSPAD Live Internal Variables out"=w351:T5)  [unwired: 6 in]
          n122 = Enqueue Element(queue=w359, element=w350) -> ()  [unwired: 2 in, 3 out]
        }
        frame "Update Image Display" {
          n123 = call "SwissSPAD Live_Next Image Acquisition Step.vi"("Error In"=w367, "Message in"=w365, "SwissSPAD Live Internal Variables in"=w370) -> ("Error Out"=w361:errorcluster, "Message out"=w366:string, "SwissSPAD Live Atomic Action"=w368:T4, "SwissSPAD Live Internal Variables out"=w369:T5)  [unwired: 5 in]
          n124 = Unbundle By Name(w370) -> ("Display Image"=w363:T1)
          n125 = call "SwissSPAD Live_Process Displayed Image.vi"("Error In"=w361, "Refnum in"=w363) -> ("Error Out"=w360:errorcluster, "Refnum out"=w362:T1)  [unwired: 8 in]
          n126 = property on="Image" class="ImageControl"(error in=w360, "Value"=w362) -> (error out=w364:errorcluster)  [unwired: 1 in, 1 out]
          n127 = Build Array(w368) -> (w371:T4[])
          n128 = Enqueue Element(queue=w372, element=w371, error in (no error)=w364) -> (error out=w375:errorcluster)  [unwired: 1 in, 2 out]
        }
        frame "Stop Live Acquisition" {
          w376 = FALSE ("Record")
          n129 = Flush Queue(queue=w384, error in (no error)=w378) -> (error out=w383:errorcluster)  [unwired: 2 out]
          n130 = call "Hide Animated Busy Icon with Message.vi"("Error In"=w383) -> ("Error Out"=w382:errorcluster)  [unwired: 10 in]
          n131 = property on="Live Button" class="Bool (strict)"("Value"=w376) -> ()  [unwired: 2 in, 2 out]
          n132 = Bundle By Name(cluster=w379, "Live Mode"=w376) -> (w377:T5)
        }
        frame "Stop Data Recording" {
          w391 = FALSE ("Record")
          n133 = Flush Queue(queue=w397) -> (error out=w396:errorcluster)  [unwired: 1 in, 2 out]
          n134 = call "Hide Animated Busy Icon with Message.vi"("Error In"=w396) -> ("Error Out"=w388:errorcluster)  [unwired: 10 in]
          n135 = Unbundle By Name(w386) -> ("Display Image"=w385:T1)
          n136 = property on="Record Button" class="Bool (strict)"("Value"=w391) -> ()  [unwired: 2 in, 2 out]
          n137 = call "Play System Sound.vi"("Windows Sound"=System_Sounds_List."notify") -> ("Error Out"=w389:errorcluster)  [unwired: 10 in]
          n138 = Bundle By Name(cluster=w386, "Current Image Set"=2147483647, "Recording Mode"=w391) -> (w395:T5)
          n139 = call <vilib>:"Clear Errors.vi"("error in (no error)"=w389) -> ()  [unwired: 5 in, 2 out]
          n140 = property on="Image" class="ImageControl"(error in=w388, "Value"=w385) -> (error out=w387:errorcluster)  [unwired: 1 in, 1 out]
        }
        frame "Stop Data Saving" {
          n141 = call "SwissSPAD Live_Abort Saving Tasks.vi"("Error In"=w404) -> ("Error Out"=w403:errorcluster, "Notebook Message"=w400:string, "UI Message"=w399:string)  [unwired: 8 in]
          n142 = call "Message Style.vi"() -> ("Message Formatting"=w405:T15)
          n143 = call "Send Message to Notebook.vi"("Text Formatting"=w405, "Error In"=w403, "Message"=w400, "Notebook Queue"=w402) -> ("Error Out"=w401:errorcluster, "Notebook Queue"=w398:refnum<queue>)  [unwired: 4 in]
        }
        frame "---- Image ----" {
        }
        frame "Copy Data to Clipboard" {
          n144 = Variant To Data(error in=w420, type=T11 {"CtlRef"=refnum, "Image to Clipboard Options"={"Include Overlay (T)"=FALSE, "Image Only (T)"=FALSE}} ("output cluster"), Variant=w421) -> (data=w417:T11, error out=w415:errorcluster)
          n145 = Unbundle(w417) -> ("CtlRef"=w416:refnum<vi>, "Image to Clipboard Options"=w413:T10)
          n146 = call "Image Display_Copy Image to Clipboard.vi"("Error In"=w415, "Image to Clipboard Options"=w413, "Display Image Control Refnum"=w416) -> ("Error Out"=w414:errorcluster)  [unwired: 8 in]
        }
        frame "Set Image Palette" {
          n147 = call "Variant to String.vi"("Variant"=w432) -> ("String"=w431:string)  [unwired: 8 in]
          n148 = call "Get User Palette Choice.vi"("Error In"=w425, "Palette"=w431) -> ("Error Out"=w429:errorcluster, "Palette Colors"=w435:u32[], "Palette Type"=w436:T13, "Palette Name (# Colors)"=w433:string)  [unwired: 3 in, 3 out]
          n149 = Bundle(cluster=T12 {"Palette Name [# Colors,int?,inv?]"="", "Palette Type"=0, "Palette Colors"=[], "Interpolate?"=FALSE} ("Image Display Palette Information"), "Palette Name [# Colors,int?,inv?]"=w433, "Palette Type"=w436, "Palette Colors"=w435) -> (w428:T12)  [unwired: 1 in]
          n150 = call "Image Display_Set Colot Palette.vi"("Error In"=w429, "Image Display Palette Information"=w428, "Display Image Control Refnum"=w427) -> ("Error Out"=w426:errorcluster)  [unwired: 8 in]
        }
        frame "Save Displayed Image with Overlay" {
          n151 = call "Image Path Dialog.vi"("error in (no error)"=w442) -> ("error out"=w445:errorcluster, "Cancelled?"=w443:bool, "Saved Image File Format"=w444:T17, "Selected Path"=w446:path, "Exists?"=w441:bool)  [unwired: 6 in]
          n152 = case shown="False" w443 {
            tunnel: w448 -> [w459 _]
            tunnel: [w458 w474] -> w447
            tunnel: w446 -> [w454 _]
            tunnel: w445 -> [w457 _]
            tunnel: w444 -> [w456 _]
            tunnel: w442 -> [_ w474]
            tunnel: w441 -> [w455 _]
            frame False {
              n153 = case shown="True" w455 {
                selector: w455 -> [w467 _]
                tunnel: w454 -> [w468 w469]
                tunnel: [w468 w469] -> w453
                tunnel: [w466 w473] -> w452
                frame False {
                  n154 = Not(x=w467) -> (.not. x?=w466:bool)
                }
                frame True {
                  n155 = Path To String(path=w469) -> (string=w471:string)
                  n156 = Format Into String(format string="%s already exists.\nOverwrite it?", w471) -> (resulting string=w470:string)  [unwired: 2 in, 1 out]
                  n157 = Two Button Dialog(message=w470) -> (T button?=w473:bool)  [unwired: 2 in]
                }
              }
              n158 = case shown="True" w452 {
                tunnel: w459 -> [_ w465]
                tunnel: [w460 w464] -> w458
                tunnel: w457 -> [w460 w463]
                tunnel: w456 -> [_ w462]
                tunnel: w453 -> [_ w461]
                frame False {
                }
                frame True {
                  n159 = call "Save Displayed Image.vi"("error in (no error)"=w463, "Saved Image File Format"=w462, "File Path in"=w461, "Display Image Control Refnum"=w465) -> ("Error Out"=w464:errorcluster)  [unwired: 6 in, 1 out]
                }
              }
            }
            frame True {
            }
          }
        }
        frame "Save Image Data as TIFF" {
          n160 = Unbundle By Name(w486) -> ("Display Image"=w485:T1)
          n161 = call "Save Image as TIFF.vi"("prompt"="Select file to save displayed SwissSPAD Live Image", "error in (no error)"=w479, "Default Name"="SwissSPAD Live Image.tif", "File Path in (Empty: Dialog)"=path "", "Image Refnum in"=w485) -> ("error out"=w482:errorcluster, "Message"=w481:string, "Cancelled?"=w480:bool)  [unwired: 3 in, 1 out]
          n162 = case shown="True" w480 {
            tunnel: [w493 w495] -> w484
            tunnel: w483 -> [w492 w494]
            tunnel: w482 -> [w491 _]
            tunnel: w481 -> [w490 _]
            tunnel: w479 -> [_ w495]
            tunnel: [w489 w494] -> w475
            frame False {
              n163 = call "Send Message to Notebook.vi"("Error In"=w491, "Message"=w490, "Notebook Queue"=w492) -> ("Error Out"=w493:errorcluster, "Notebook Queue"=w489:refnum<queue>)  [unwired: 5 in]
            }
            frame True {
            }
          }
        }
      }
      n164 = local write "Message"(w80) -> ()
      n165 = call "SwissSPAD Live_Filter Error.vi"("error in (no error)"=w70, "SS2 Q Elements in"=w69) -> ("error out"=w68:errorcluster, "SS2 Q Elements out"=w67:T4[])  [unwired: 8 in]
      n166 = call "SwissSPAD Live_Update Buttons.vi"("SwissSPAD Live Internal Variables in"=w74) -> ("SwissSPAD Live Internal Variables out"=w76:T5)  [unwired: 6 in]
      n167 = Empty Array?(array=w67) -> (empty?=w87:bool)
    }
    n168 = call "SwissSPAD Live_Internal Variables Storage.vi"("Set/Get(F)"=TRUE, "Error In"=w44, "SwissSPAD Live Internal Variables in"=w58) -> ("Error Out"=w43:errorcluster, "SwissSPAD Live Internal Variables"=w46:T5)  [unwired: 7 in]
    n169 = call "Send Error to Notebook.vi"("error in (no error)"=w43, "State Machine Case Error Source"=w53, "Notebook Q"=w56) -> ("Error Out"=w55:errorcluster)  [unwired: 8 in]
    n170 = call "Clear Error.vi"("Error In"=w55) -> ("no Error Out"=w54:errorcluster)  [unwired: 8 in]
  }
  n171 = while {
    tunnel: w29 -> [w498]
    tunnel: w18 -> [_]
    tunnel: w17 -> [w497]
    tunnel: w16 -> [w496]
    stop <- w499 stop-if-true
    # "Event Loop"
    n172 = event shown="[3] \"Record Button\": Value Change" {
      selector: _ -> [_ _ _ _ _ _ _ _ _ _]
      dyn-events: _ -> [_ _ _ _ _ _ _ _ _ _]
      timeout: _ -> [_ _ _ _ _ _ _ _ _ _]
      tunnel: [w504 w515 _ _ _ TRUE _ _ _ _] -> w499
      tunnel: w498 -> [w508 w516 w555 w571 _ w597 w598 w630 _ w646]
      tunnel: w497 -> [_ _ _ _ _ _ _ _ w639 _]
      tunnel: w496 -> [_ _ _ _ _ _ _ _ w638 _]
      event Panel Close? {
        n173 = event-data() -> ()  [unwired: 1 in, 1 out]
        n174 = local read "Record Button"() -> (w506:bool)
        n175 = local read "Live Button"() -> (w507:bool)
        n176 = call "SwissSPAD Live_Internal Data Storage.vi"("SS2 Live Data"=SwissSPAD_Live_Internal_Data_List."Number of pending file saving tasks") -> ("Variant"=w501:variant)  [unwired: 8 in, 2 out]
        n177 = call "Variant to I32.vi"("Variant"=w501) -> ("Value"=w500:i32)  [unwired: 8 in]
        n178 = Not Equal To 0?(x=w500) -> (x != 0?=w505:bool)
        n179 = Build Array(w507, w506, w505) -> (w503:bool[])
        n180 = call "SwissSPAD Live_Ready to Quit.vi"("Flags"=w503, "SS2 Live Queue in"=w508) -> ("Ready to Quit?"=w504:bool)  [unwired: 8 in, 1 out]
        n181 = event-data("Discard?"=TRUE) -> ()  [unwired: 1 in, 1 out]
      }
      event Menu Selection (User) {
        n182 = event-data() -> ("ItemTag"=w517:string)  [unwired: 1 in]
        n183 = call "SwissSPAD Live_Internal Variables Storage.vi"("Set/Get(F)"=FALSE) -> ("SwissSPAD Live Internal Variables"=w514:T5)  [unwired: 9 in, 1 out]
        n184 = Unbundle By Name(w514) -> ("Recording Mode"=w513:bool, "Live Mode"=w512:bool)
        n185 = Or(x=w513, y=w512) -> (x .or. y?=w511:bool)
        n186 = case shown="\"Reset FPGA(s)\"" w517 {
          tunnel: w516 -> [_ _ w524 _ _ _ _ _ w538 w542 w546 _ _]
          tunnel: [_ _ w523 _ _ _ _ _ _ _ _ _ _] -> w515
          tunnel: w511 -> [_ _ _ _ _ _ _ _ w537 w541 w545 _ _]
          frame "", Default {
          }
          frame "------ File -------" {
          }
          frame "Quit" {
            n187 = local read "Record Button"() -> (w526:bool)
            n188 = local read "Live Button"() -> (w525:bool)
            n189 = call "SwissSPAD Live_Internal Data Storage.vi"("SS2 Live Data"=SwissSPAD_Live_Internal_Data_List."Number of pending file saving tasks") -> ("Variant"=w519:variant)  [unwired: 8 in, 2 out]
            n190 = call "Variant to I32.vi"("Variant"=w519) -> ("Value"=w518:i32)  [unwired: 8 in]
            n191 = Not Equal To 0?(x=w518) -> (x != 0?=w521:bool)
            n192 = Build Array(w525, w526, w521) -> (w522:bool[])
            n193 = call "SwissSPAD Live_Ready to Quit.vi"("Flags"=w522, "SS2 Live Queue in"=w524) -> ("Ready to Quit?"=w523:bool)  [unwired: 8 in, 1 out]
          }
          frame "----- Windows -------" {
          }
          frame "Settings" {
            n194 = call "SwissSPAD Live_Get Ancillary Window Path.vi"("SS2 Live Windows"=SwissSPAD_Live_Windows_List."Settings Window") -> ("Error Out"=w527:errorcluster, "VI Path"=w528:path)  [unwired: 9 in]
            n195 = call "Run Vi.vi"("VI Path"=w528, "error in (no error)"=w527) -> ()  [unwired: 6 in, 2 out]
          }
          frame "Histogram" {
            n196 = call "SwissSPAD Live_Get Ancillary Window Path.vi"("SS2 Live Windows"=SwissSPAD_Live_Windows_List."Histogram Window") -> ("Error Out"=w530:errorcluster, "VI Path"=w531:path)  [unwired: 9 in]
            n197 = call "Run Vi.vi"("VI Path"=w531, "error in (no error)"=w530) -> ()  [unwired: 6 in, 2 out]
          }
          frame "Notebook" {
            n198 = call "SwissSPAD Live_Get Ancillary Window Path.vi"("SS2 Live Windows"=SwissSPAD_Live_Windows_List."Notebook Window") -> ("Error Out"=w534:errorcluster, "VI Path"=w535:path)  [unwired: 9 in]
            n199 = call "Run Vi.vi"("VI Path"=w535, "error in (no error)"=w534, "Start Hidden? (F)"=TRUE) -> ()  [unwired: 5 in, 2 out]
          }
          frame "----- Hardware ------" {
          }
          frame "Connect to FPGA(s)" {
            n200 = case shown="False" w537 {
              tunnel: w538 -> [w540 _]
              frame False {
                n201 = Enqueue Element(queue=w540, element=T4[] [{"SwissSPAD Q Event"=enum."Init FPGA(s)", "Data"=variant}]) -> ()  [unwired: 2 in, 3 out]
              }
              frame True {
              }
            }
          }
          frame "FPGA(s) Status" {
            n202 = case shown="False" w541 {
              tunnel: w542 -> [w544 _]
              frame False {
                n203 = Enqueue Element(queue=w544, element=T4[] [{"SwissSPAD Q Event"=enum."FPGA(s) Status", "Data"=variant}]) -> ()  [unwired: 2 in, 3 out]
              }
              frame True {
              }
            }
          }
          frame "Reset FPGA(s)" {
            n204 = case shown="False" w545 {
              tunnel: w546 -> [w548 _]
              frame False {
                n205 = Enqueue Element(queue=w548, element=T4[] [{"SwissSPAD Q Event"=enum."Reset FPGA(s)", "Data"=variant}]) -> ()  [unwired: 2 in, 3 out]
              }
              frame True {
              }
            }
          }
          frame "------- Help -------" {
          }
          frame "About" {
            n206 = call "SwissSPAD Live_Get Ancillary Window Path.vi"("SS2 Live Windows"=SwissSPAD_Live_Windows_List."About Window") -> ("Error Out"=w549:errorcluster, "VI Path"=w550:path)  [unwired: 9 in]
            n207 = call "Run Vi.vi"("VI Path"=w550, "error in (no error)"=w549) -> ()  [unwired: 6 in, 2 out]
          }
        }
      }
      event "Live Button": Value Change {
        n208 = event-data() -> ("OldVal"=w552:bool)  [unwired: 1 in]
        n209 = local read "Record Button"() -> (w553:bool)
        n210 = case shown="False" w553 {
          tunnel: w555 -> [w557 _]
          tunnel: "Live Button" -> [w556 _]
          tunnel: w552 -> [_ w566]
          frame False {
            n211 = case shown="False" w556 {
              tunnel: w557 -> [w562 w565]
              frame False {
                n212 = Flush Queue(queue=w562) -> (queue out=w560:refnum<queue>, error out=w559:errorcluster)  [unwired: 1 in, 1 out]
                n213 = Build Array(T4 {"SwissSPAD Q Event"=enum."Stop Live Acquisition", "Data"=variant} ("element")) -> (w561:T4[])
                n214 = Enqueue Element At Opposite End(queue=w560, element=w561, error in (no error)=w559) -> ()  [unwired: 1 in, 3 out]
              }
              frame True {
                n215 = Build Array(T4 {"SwissSPAD Q Event"=enum."Start Live Acquisition", "Data"=variant} ("element")) -> (w563:T4[])
                n216 = Enqueue Element(queue=w565, element=w563) -> ()  [unwired: 2 in, 3 out]
              }
            }
          }
          frame True {
            n217 = property on="Live Button" class="Bool (strict)"("Value"=w566) -> ()  [unwired: 2 in, 2 out]
            n218 = One Button Dialog(message="Recording in progress: wait or abort before switching to Live Mode") -> ()  [unwired: 1 in, 1 out]
          }
        }
      }
      event "Record Button": Value Change {
        n219 = event-data() -> ("OldVal"=w568:bool)  [unwired: 1 in]
        n220 = local read "Live Button"() -> (w569:bool)
        n221 = case shown="False" w569 {
          tunnel: w571 -> [w573 _]
          tunnel: "Record Button" -> [w572 _]
          tunnel: w568 -> [_ w586]
          frame False {
            n222 = case shown="True" w572 {
              selector: w572 -> [_ w580]
              tunnel: w573 -> [w578 w584]
              frame False {
                n223 = Flush Queue(queue=w578) -> (queue out=w576:refnum<queue>, error out=w575:errorcluster)  [unwired: 1 in, 1 out]
                n224 = Build Array(T4 {"SwissSPAD Q Event"=enum."Stop Data Recording", "Data"=variant} ("element")) -> (w577:T4[])
                n225 = Enqueue Element At Opposite End(queue=w576, element=w577, error in (no error)=w575) -> ()  [unwired: 1 in, 3 out]
              }
              frame True {
                n226 = disable-structure shown="Disabled" {
                  disable-tunnel: [T4 {"SwissSPAD Q Event"=enum."Reset FPGA(s)", "Data"=variant} ("element") _] -> w579
                  frame Disabled {
                  }
                  frame Enabled {
                  }
                }
                n227 = Bundle By Name(cluster=T4 {"SwissSPAD Q Event"=enum."Start Recording", "Data"=variant} ("element"), "Data"=w580) -> (w581:T4)
                n228 = Build Array(w579, w581) -> (w582:T4[])
                n229 = Enqueue Element(queue=w584, element=w582) -> ()  [unwired: 2 in, 3 out]
              }
            }
          }
          frame True {
            n230 = property on="Record Button" class="Bool (strict)"("Value"=w586) -> ()  [unwired: 2 in, 2 out]
            n231 = One Button Dialog(message="Live mode on: Stop before switching to Recording Mode") -> ()  [unwired: 1 in, 1 out]
          }
        }
      }
      event "Abort": Value Change {
        n232 = event-data() -> ()  [unwired: 1 in, 6 out]
        n233 = global write "SwissSPAD Live_Globals.vi" "Abort"("Abort") -> ()
      }
      event Application Instance Close {
        n234 = event-data() -> ()  [unwired: 1 in, 1 out]
        n235 = Flush Queue(queue=w597) -> (queue out=w593:refnum<queue>)  [unwired: 1 in, 2 out]
        n236 = local read "Live Button"() -> (w592:bool)
        n237 = Select(t=T4 {"SwissSPAD Q Event"=enum."Stop Live Acquisition", "Data"=variant} ("element"), s=w592, f=T4 {"SwissSPAD Q Event"=enum."Stop Data Recording", "Data"=variant} ("element")) -> (s? t:f=w589:T4)
        n238 = Build Array(w589, T4 {"SwissSPAD Q Event"=enum."Quit", "Data"=variant} ("element")) -> (w594:T4[])
        n239 = Enqueue Element(queue=w593, element=w594) -> ()  [unwired: 2 in, 3 out]
      }
      event "Image": Shortcut Menu Selection (User) {
        n240 = event-data() -> ("ItemTag"=w600:string, "CtlRef"=w599:refnum<vi>)  [unwired: 1 in]
        n241 = case shown="\"Save Image Data as TIFF\"" w600 {
          selector: w600 -> [_ _ _ w615 _ _ _ _]
          tunnel: w599 -> [_ w603 w610 _ _ _ w627 w629]
          tunnel: w598 -> [_ w607 w614 w619 w622 w625 _ _]
          frame "", Default {
          }
          frame "Copy Data to Clipboard" {
            n242 = Bundle("CtlRef"=w603, "Image to Clipboard Options"=T10 {"Include Overlay (T)"=TRUE, "Image Only (T)"=FALSE}) -> (w601:T11)  [unwired: 1 in]
            n243 = Bundle By Name(cluster=T4 {"SwissSPAD Q Event"=enum."Copy Data to Clipboard", "Data"=variant} ("SS2 Q Element"), "Data"=w601) -> (w605:T4)
            n244 = Build Array(w605) -> (w604:T4[])
            n245 = Enqueue Element(queue=w607, element=w604) -> ()  [unwired: 2 in, 3 out]
          }
          frame "Copy Image Only (with Overlay)" {
            n246 = Bundle("CtlRef"=w610, "Image to Clipboard Options"=T10 {"Include Overlay (T)"=TRUE, "Image Only (T)"=TRUE}) -> (w608:T11)  [unwired: 1 in]
            n247 = Bundle By Name(cluster=T4 {"SwissSPAD Q Event"=enum."Copy Data to Clipboard", "Data"=variant} ("SS2 Q Element"), "Data"=w608) -> (w612:T4)
            n248 = Build Array(w612) -> (w611:T4[])
            n249 = Enqueue Element(queue=w614, element=w611) -> ()  [unwired: 2 in, 3 out]
          }
          frame "Binary", "Gradient", "Grayscale", "Rainbow", "Temperature" {
            n250 = Bundle By Name(cluster=T4 {"SwissSPAD Q Event"=enum."Set Image Palette", "Data"=variant} ("SS2 Q Element"), "Data"=w615) -> (w617:T4)
            n251 = Build Array(w617) -> (w616:T4[])
            n252 = Enqueue Element(queue=w619, element=w616) -> ()  [unwired: 2 in, 3 out]
          }
          frame "Save Displayed Image with Overlay" {
            n253 = Build Array(T4 {"SwissSPAD Q Event"=enum."Save Displayed Image with Overlay", "Data"=variant} ("SS2 Q Element")) -> (w621:T4[])
            n254 = Enqueue Element(queue=w622, element=w621) -> ()  [unwired: 2 in, 3 out]
          }
          frame "Save Image Data as TIFF" {
            n255 = Build Array(T4 {"SwissSPAD Q Event"=enum."Save Image Data as TIFF", "Data"=variant} ("SS2 Q Element")) -> (w624:T4[])
            n256 = Enqueue Element(queue=w625, element=w624) -> ()  [unwired: 2 in, 3 out]
          }
          frame "Zoom to Fit" {
            n257 = call "Image Display_Zoom to Fit.vi"("Keep Aspect Ratio (T)"=FALSE, "Display Image Control Refnum"=w627) -> ()  [unwired: 9 in, 1 out]
          }
          frame "Zoom to Fit (Keep Aspect Ratio)" {
            n258 = call "Image Display_Zoom to Fit.vi"("Keep Aspect Ratio (T)"=TRUE, "Display Image Control Refnum"=w629) -> ()  [unwired: 9 in, 1 out]
          }
        }
      }
      event "Saving in progress": Shortcut Menu Selection (User) {
        n259 = event-data() -> ("ItemTag"=w631:string)  [unwired: 1 in]
        n260 = case shown="\"Abort All Saving Tasks\"" w631 {
          tunnel: w630 -> [_ w633]
          frame "", Default {
          }
          frame "Abort All Saving Tasks" {
            n261 = property on="Record Button" class="Bool (strict)"() -> ("Value"=w632:bool)  [unwired: 2 in, 2 out]
            n262 = case shown="False" w632 {
              tunnel: w633 -> [w635 _]
              frame False {
                n263 = Enqueue Element(queue=w635, element=T4[] [{"SwissSPAD Q Event"=enum."Stop Data Saving", "Data"=variant}]) -> ()  [unwired: 2 in, 3 out]
              }
              frame True {
                n264 = One Button Dialog(message="Please first abort Recording Task.") -> ()  [unwired: 1 in, 1 out]
              }
            }
          }
        }
      }
      event "Image": Mouse Up {
        n265 = event-data() -> ("CtlRef"=w644:refnum<vi>)  [unwired: 1 in]
        n266 = property class="ImageControl"(reference=w644) -> (error out=w642:errorcluster, "ROI"=w643:T19)  [unwired: 1 in, 1 out]
        n267 = call "SwissSPAD Live_Internal Data Storage.vi"("Get(F)/Set"=TRUE, "SS2 Live Data"=SwissSPAD_Live_Internal_Data_List."Current Image ROI Information", "Error In"=w642, "Variant"=w643) -> ("Error Out"=w637:errorcluster)  [unwired: 5 in, 2 out]
        n268 = call "SwissSPAD Live_Update Image Information Event.vi"("error in (no error)"=w637, "Calling VI Name"=w638, "User Event in"=w639) -> ()  [unwired: 9 in]
      }
      event "Refresh": Value Change {
        n269 = event-data() -> ()  [unwired: 1 in, 1 out]
        n270 = Enqueue Element(queue=w646, element=T4[] [{"SwissSPAD Q Event"=enum."Refresh Display Image", "Data"=variant}]) -> ()  [unwired: 2 in, 3 out]
      }
    }
  }
  n271 = while {
    tunnel: w21 -> [w648]
    stop <- w647 stop-if-true
    n272 = event shown="[0] Timeout" {
      selector: w648 -> [_ w664]
      dyn-events: _ -> [_ _]
      timeout: 100 -> [_ _]
      tunnel: [_ TRUE] -> w647
      event Timeout {
        n273 = event-data() -> ()  [unwired: 1 in, 1 out]
        n274 = call "SwissSPAD Live_Get-Set Saving Tasks Information.vi"() -> ("error out"=w650:errorcluster, "# Saving Tasks"=w652:i32, "Array of Saving Tasks Information"=w651:T20[])  [unwired: 8 in, 1 out]
        n275 = case shown="0" w652 {
          tunnel: w651 -> [_ w662]
          tunnel: w650 -> [_ w658]
          frame 0 {
            n276 = property on="Saving in progress" class="Bool (strict)"() -> ("Visible"=w653:bool)  [unwired: 2 in, 2 out]
            n277 = case shown="False" w653 {
              frame False {
              }
              frame True {
                n278 = call "Play System Sound.vi"("Windows Sound"=System_Sounds_List."tada") -> ("Error Out"=w655:errorcluster)  [unwired: 10 in]
                n279 = call <vilib>:"Clear Errors.vi"("error in (no error)"=w655) -> ("error out"=w654:errorcluster)  [unwired: 5 in, 1 out]
                n280 = property on="Saving in progress" class="Bool (strict)"(error in=w654, "Visible"=FALSE) -> ()  [unwired: 1 in, 2 out]
              }
            }
          }
          frame 1, Default {
            w660 = TRUE ("Saving in progress")
            n281 = call "SwissSPAD Live_Saving Tasks Description.vi"("Error In"=w658, "Array of Saving Tasks Information"=w662) -> ("Error Out"=w659:errorcluster, "Description"=w661:string)  [unwired: 8 in]
            n282 = property on="Saving in progress" class="Bool (strict)"(error in=w659, "Value"=w660, "Blinking"=w660, "Visible"=w660, "Desc"=w661) -> ()  [unwired: 1 in, 2 out]
          }
        }
      }
      event User Event {
        n283 = event-data() -> ("UsrEvtRef"=w666:refnum<user-event>)  [unwired: 1 in]
        n284 = Unregister For Events(event registration refnum=w664) -> (error out=w663:errorcluster)  [unwired: 1 in]
        n285 = Destroy User Event(user event=w666, error in=w663) -> ()  [unwired: 1 out]
      }
    }
  }
  n286 = case shown="True" TRUE {
    frame False {
    }
    frame True {
    }
  }
  n287 = case shown="False" w41 {
    tunnel: w39 -> [_ w667]
    frame False {
    }
    frame True {
      n288 = invoke class="VI" method="FP.Close"(reference=w667) -> ()  [unwired: 2 in, 3 out]
    }
  }
  n289 = Release Queue(queue=w29, force destroy? (F)=w25, error in (no error)=w5) -> ()  [unwired: 3 out]
  n290 = Release Queue(queue=w23, force destroy? (F)=w25, error in (no error)=w5) -> ()  [unwired: 3 out]
  n291 = call "SwissSPAD Live_Exit Cleanup.vi"("Error In"=w5, "SwissSPAD Live Internal Variables"=w33) -> ("Error Out"=w4:errorcluster)  [unwired: 9 in]
  n292 = for {
    tunnel: w6 -> [w669] mode=indexing
    tunnel: w4 -> [_]
    tunnel: [w668] -> w3 mode=indexing
    n293 = call "SwissSPAD Live_Get Ancillary Window Path.vi"("SS2 Live Windows"=w669) -> ("VI Path"=w668:path)  [unwired: 9 in, 1 out]
  }
  n294 = call "Close & Abort VIs.vi"("Abort (T)"=FALSE, "VI Paths"=w3) -> ("Error Out"=w1:errorcluster)  [unwired: 9 in]
  n295 = call "Clear Error.vi"("Error In"=w1) -> ()  [unwired: 8 in, 1 out]
  "Bottom FPGA Status" <- w7
  "Top FPGA Status" <- w7
